vi "PSO_Create Population.vi"(5 "Function Data":variant, 6 "Parameters":T1={"Swarm size"=100, "Generations no."=500, "Cognitive coeff a1"=6.0, "Social coeff a2"=0.85, "Min inertia weight"=0.0, "Max inertia weight "=0.9, "Fmax"=0} {"Generations no." min=1; "Swarm size" min=1}, 7 "Fitness Function":T3, 8 "Phenotype size":i32, 9 "Population size":i32) -> (3 "Population out":T2)   [LabVIEW 2016, in "Optimal Frequency Bands Search.lvlib" / "ParticleSwarm.lvlib"]
doc: "Создать рой частиц. Начальные координаты частиц задаются случайным образом."
uses:
  ParticleSwarm.lvlib
  tFitness Function.ctl
  PSO_tPopulation.ctl
  PSO_tParameters.ctl
  <vilib>/gmath/statdist.llb/Uniform (Discrete) Random.vi
  <vilib>/gmath/NI_Gmath.lvlib
panel:
  # "This VI is a part of BCI Design library, http://www.ru-bci.org \nCopyright © 2020, Sotnikov Peter, All rights reserved. License: CC BY-NC 4.0"
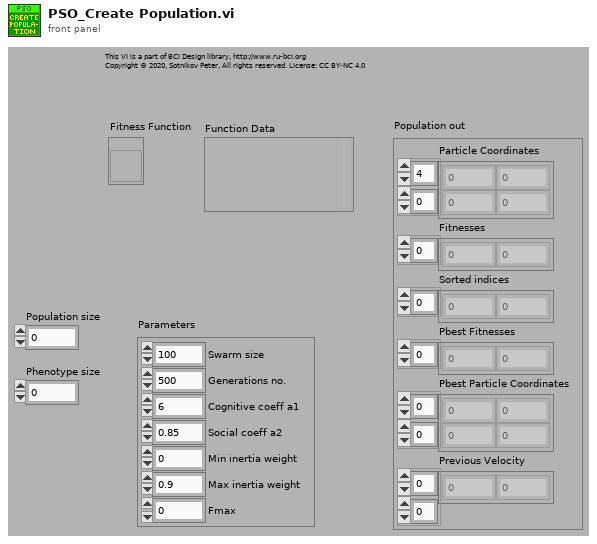
[diagram p1: front panel]
types:
  T1 = typedef "Optimal Frequency Bands Search.lvlib/ParticleSwarm.lvlib/PSO_tParameters.ctl" = cluster{"Swarm size":i32, "Generations no.":i32, "Cognitive coeff a1":dbl, "Social coeff a2":dbl, "Min inertia weight":dbl, "Max inertia weight ":dbl, "Fmax":i32}
  T2 = typedef "Optimal Frequency Bands Search.lvlib/ParticleSwarm.lvlib/PSO_tPopulation.ctl" = cluster{"Particle Coordinates":i32[][], "Fitnesses":dbl[], "Sorted indices":i32[], "Pbest Fitnesses":dbl[], "Pbest Particle Coordinates":i32[][], "Previous Velocity":dbl[][]}
  T3 = typedef "Optimal Frequency Bands Search.lvlib/ParticleSwarm.lvlib/tFitness Function.ctl" = refnum<vi>
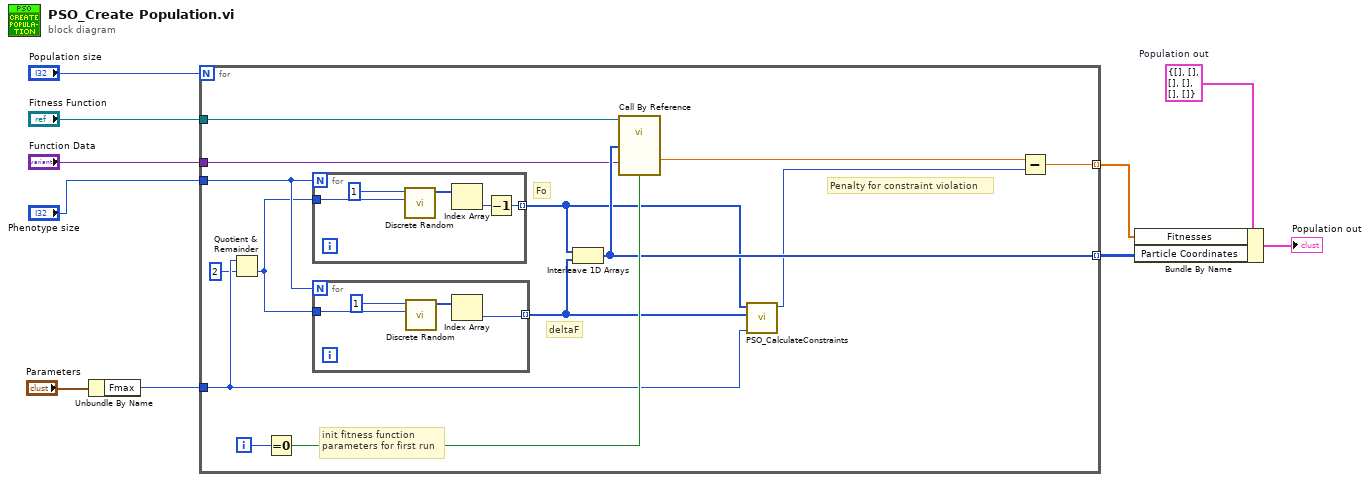
[diagram p0: block diagram]
diagram:
  w10 = T2 {"Particle Coordinates"=[], "Fitnesses"=[], "Sorted indices"=[], "Pbest Fitnesses"=[], "Pbest Particle Coordinates"=[], "Previous Velocity"=[]}  # Population out
  n1 = Unbundle By Name("Parameters") -> ("Fmax"=w1:i32)
  n2 = for {
    N: "Population size" -> [_]
    tunnel: [w18] -> w3 mode=indexing
    tunnel: [w22] -> w4 mode=indexing
    tunnel: "Fitness Function" -> [w21]
    tunnel: "Function Data" -> [w20]
    tunnel: "Phenotype size" -> [w19]
    tunnel: w1 -> [w14]
    i -> [w24]
    # "Penalty for constraint violation"
    # "deltaF"
    # "Fo"
    # "init fitness function\nparameters for first run"
    n3 = Quotient & Remainder(x=w14, y=2) -> (floor(x/y)=w12:i32)  [unwired: 1 out]
    n4 = Equal To 0?(x=w24) -> (x = 0?=w23:bool)
    n5 = for {
      N: w19 -> [_]
      tunnel: [w30] -> w17 mode=indexing
      tunnel: w12 -> [w29]
      n6 = call-poly <vilib>:"Discrete Random.vi"("n"=w29, "samples"=1) -> ("uniform (discrete) random data"=w32:i32[])  [unwired: 8 in, 1 out]
      n7 = Index Array(array=w32) -> (element=w31:i32)  [unwired: 1 in]
      n8 = Decrement(x=w31) -> (x-1=w30:i32)
    }
    n9 = for {
      N: w19 -> [_]
      tunnel: [w26] -> w16 mode=indexing
      tunnel: w12 -> [w25]
      n10 = call-poly <vilib>:"Discrete Random.vi"("n"=w25, "samples"=1) -> ("uniform (discrete) random data"=w27:i32[])  [unwired: 8 in, 1 out]
      n11 = Index Array(array=w27) -> (element=w26:i32)  [unwired: 1 in]
    }
    n12 = Interleave 1D Arrays(w17, w16) -> (w22:i32[])
    n13 = call-by-ref "Call By Reference"(reference=w21, "Init? (F)"=w23, "Data"=w20, "Phenotype"=w22) -> ("Fitness"=w11:dbl)  [unwired: 1 in, 2 out]
    n14 = call "PSO_CalculateConstraints.vi"("Fmax"=w14, "deltaF vector"=w16, "F0 vector"=w17) -> ("Penalty"=w15:i32)  [unwired: 7 in, 1 out]
    n15 = Subtract(x=w11, y=w15) -> (x-y=w18:dbl)
  }
  n16 = Bundle By Name(cluster=w10, "Fitnesses"=w3, "Particle Coordinates"=w4) -> (→"Population out":T2)
